vi "Update Fan Status.vi"(8 "error in (no error)":errorcluster, 9 "Fan B":T1, 10 "Fan A":T1, 11 "Cooler UI in":refnum<class "Live User Controller.lvclass">) -> (0 "error out":errorcluster, 3 "Cooler UI out":refnum<class "Live User Controller.lvclass">)   [LabVIEW 2025, in "Live User Controller.lvclass"]
doc: "Update the user interface to show the fan status."
uses:
  Live User Controller.lvclass
  Dual Fan/Dual Fan/Fan Info.ctl
  Live User Controller.lvclass/Live User Controller.ctl
  Dual Fan/Dual Fan/Dual Fan.lvclass
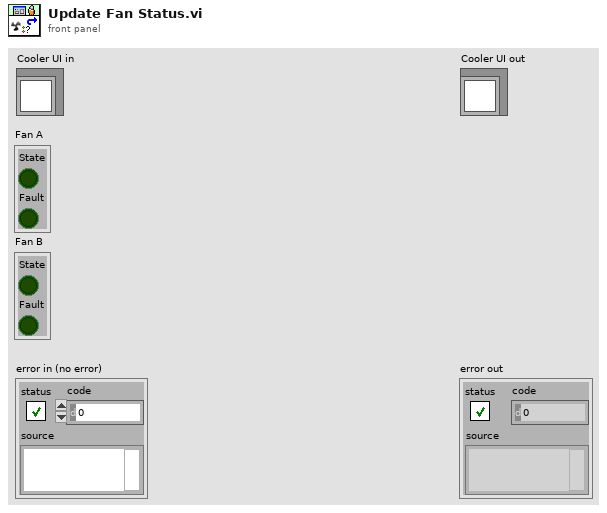
[diagram p1: front panel]
types:
  T1 = typedef "Dual Fan.lvlib/Dual Fan.lvclass/Fan Info.ctl" = cluster{"State":bool, "Fault":bool}
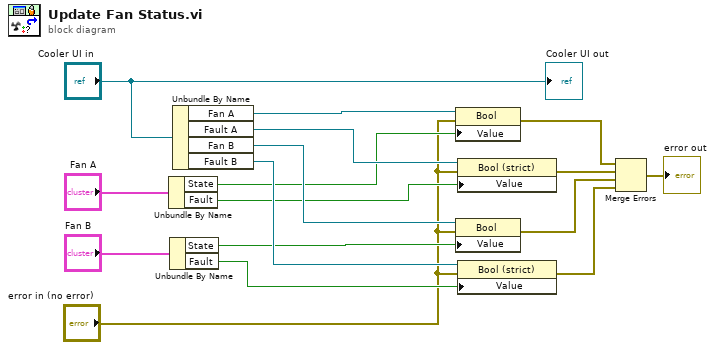
[diagram p0: block diagram]
diagram:
  n1 = Unbundle By Name("Fan A") -> ("State"=w9:bool, "Fault"=w10:bool)
  n2 = Unbundle By Name("Fan B") -> ("State"=w8:bool, "Fault"=w11:bool)
  n3 = Unbundle By Name("Cooler UI in") -> ("Fan A"=w17:refnum<vi>, "Fault A"=w16:refnum<vi>, "Fan B"=w15:refnum<vi>, "Fault B"=w14:refnum<vi>)
  n4 = property class="Bool"(reference=w17, error in="error in (no error)", "Value"=w9) -> (error out=w6:errorcluster)  [unwired: 1 out]
  n5 = property class="Bool"(reference=w15, error in="error in (no error)", "Value"=w8) -> (error out=w4:errorcluster)  [unwired: 1 out]
  n6 = property class="Bool (strict)"(reference=w16, error in="error in (no error)", "Value"=w10) -> (error out=w5:errorcluster)  [unwired: 1 out]
  n7 = property class="Bool (strict)"(reference=w14, error in="error in (no error)", "Value"=w11) -> (error out=w3:errorcluster)  [unwired: 1 out]
  n8 = Merge Errors(w6, w5, w4, w3) -> (→"error out":errorcluster)
  "Cooler UI out" <- "Cooler UI in"
